vi "microspec_validating_v9.vi"() -> ()   [LabVIEW 2013]
uses:
  <vilib>/Instr/_visa.llb/VISA Configure Serial Port (Instr).vi
  <vilib>/Utility/file.llb/Write To Spreadsheet File (string).vi
panel:
  in  "Path":path
  in  "intergration time":dbl=54.0 caption="sensor\nintergration time (us)" min=54.0 max=5000000.0 step=100.0
  in  "?":T1(tab)=enum."measuring sequence"
  out "radiometer data file path":path
  in  "Runname":string
  out "Sensor_name":string="ILT1400"
  out "Radiometer Average":dbl
  in  "Delay":dbl=1.0
  in  "Step":dbl=1.0
  in  "Stop Wl":dbl=900.0 min=0.0 max=5000.0 step=100.0
  in  "Start Wl":dbl=300.0 min=0.0 max=5000.0 step=100.0
  in  "mean_number":i32=1 caption="Mean Number"
  out "Current Wavelength":dbl
  out "XY-Graph 2":cluster{"Y":dbl[], "Y":dbl[]}[](graph)
  in  "run 5":bool
  out "sectrometer data file path":path
  in  "save data":bool
  in  "reset with every wavelength?":bool caption="reset with new run?"
  in  "Delay":dbl=1.0
  in  "Step":dbl=10.0
  in  "Stop Wl":dbl=900.0 min=0.0 max=5000.0 step=100.0
  out "Current Wavelength":dbl
  in  "Start Wl 2":dbl=300.0 min=0.0 max=5000.0 step=10.0
  in  "Sensor":string(combo)="C12880MA_15B00040"
  in  "run 2":bool
  in  "Set Runs":i32=1
  out "Current Run":i32
  in  "stop runs":bool
  out "raw_data":cluster{"Y":dbl[], "Y":dbl[]}[](graph) caption="raw data"
  out "raw_data 2":cluster{"Y":dbl[], "Y":dbl[]}[](graph) caption="raw data"
  in  "Stopp":bool
  out "System Setup":i32
  out "DLL Version":string
  out "Get Version":i32
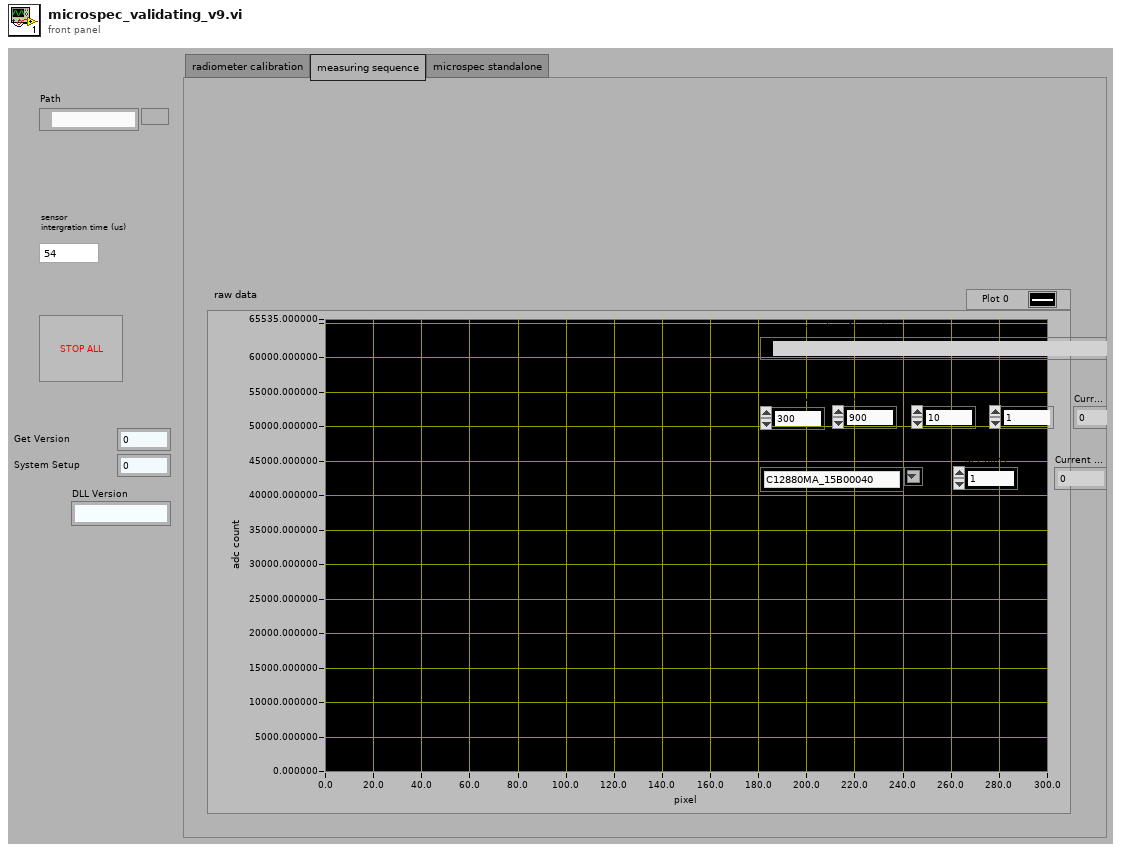
[diagram p1: front panel]
types:
  T1 = enum32{"radiometer calibration", "measuring sequence", "microspec standalone"}
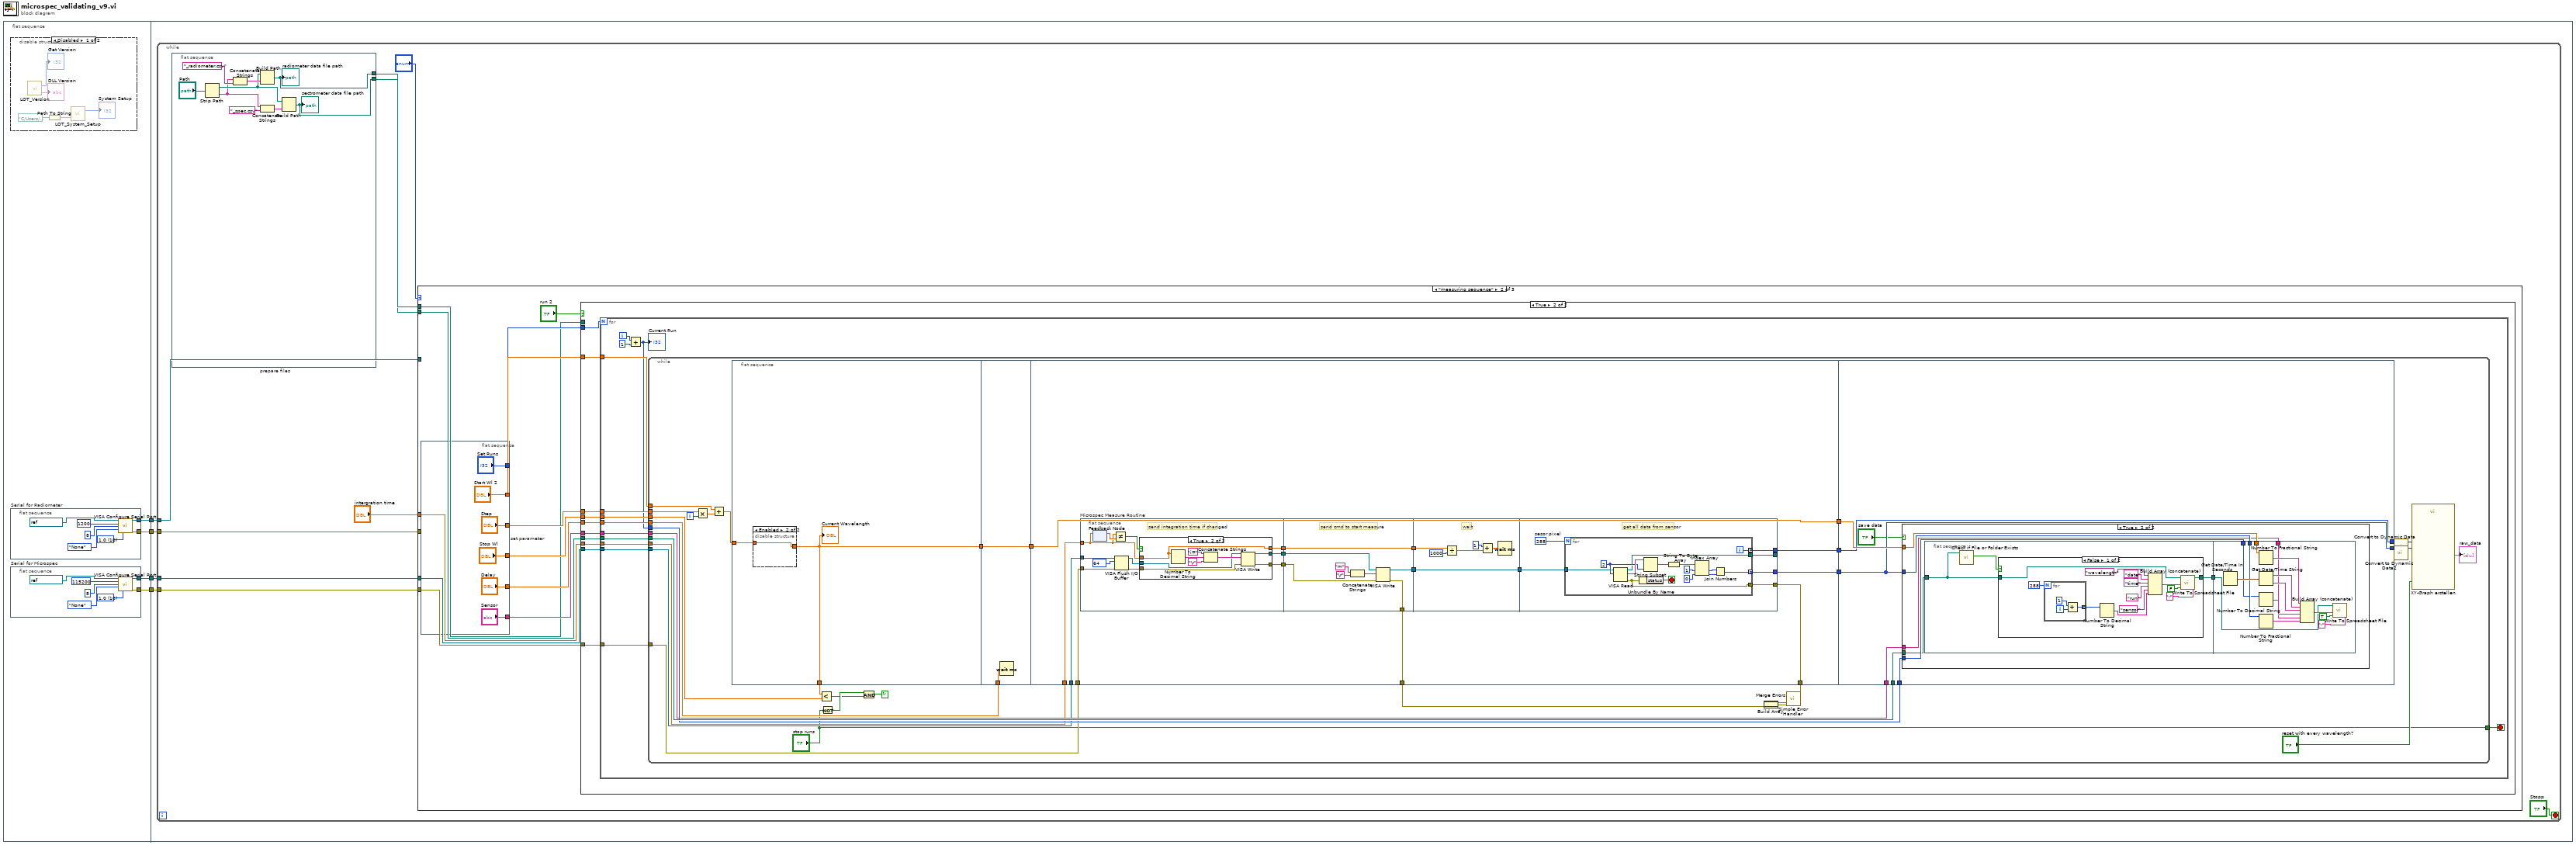
[diagram p0: block diagram]
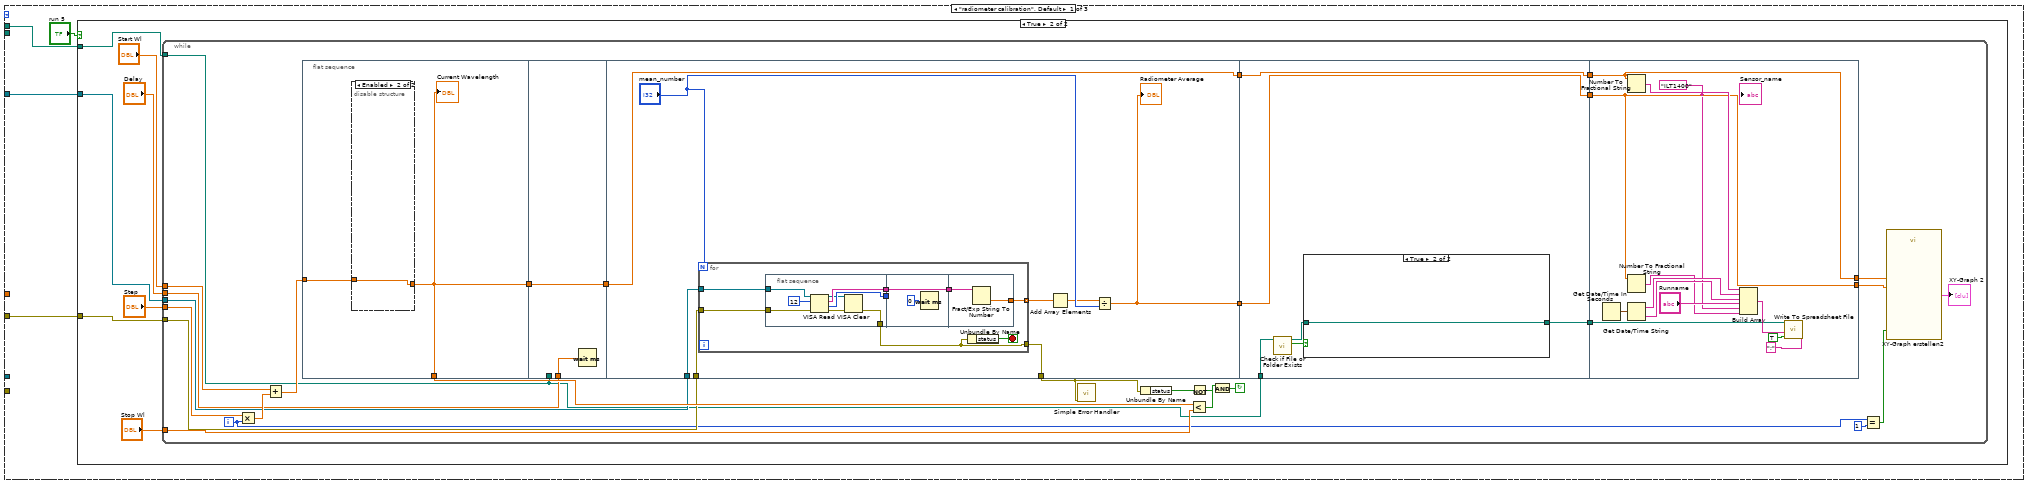
[diagram p3: hidden frame]
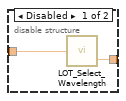
[diagram p5: hidden frame]
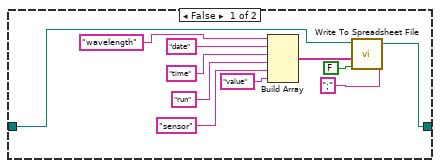
[diagram p6: hidden frame]
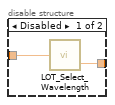
[diagram p8: hidden frame]
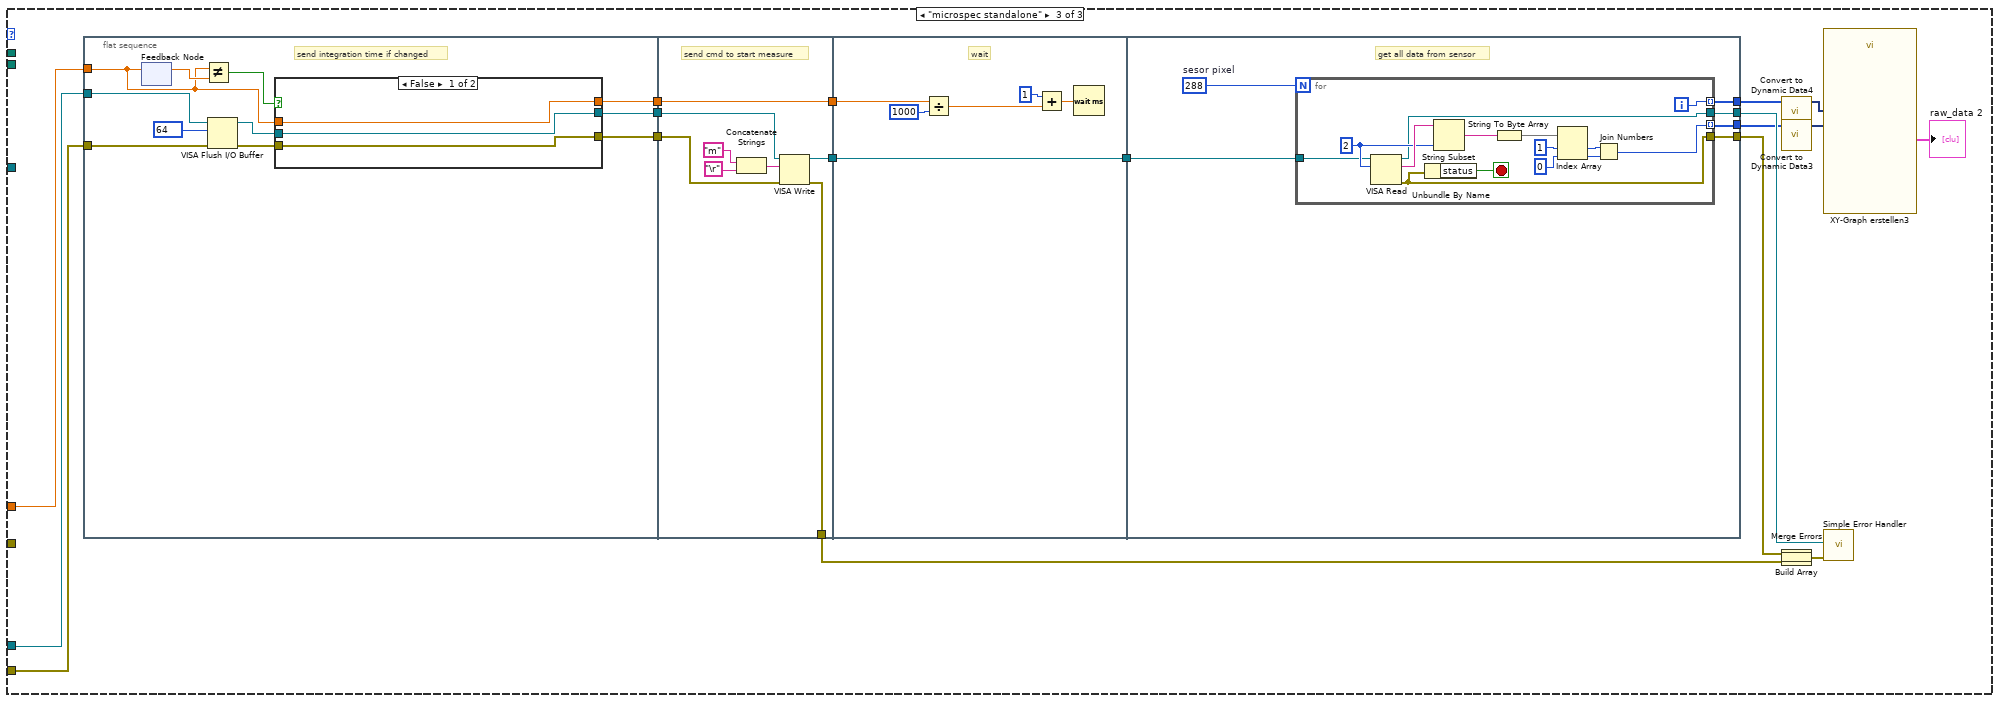
[diagram p12: hidden frame]
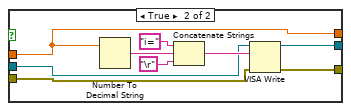
[diagram p13: hidden frame]
diagram:
  n1 = flat-sequence {
    tunnel: [w8] -> w4
    tunnel: [w7] -> w3
    tunnel: [w6] -> w2
    tunnel: [w5] -> w1
    tunnel: w4 -> [w31]
    tunnel: w3 -> [w30]
    tunnel: w2 -> [w29]
    tunnel: w1 -> [w28]
    frame #0 {
      # "Configuration"
      n2 = disable-structure shown="Disabled" {
        frame Disabled {
          n3 = call "LOT_Version.vi"() -> ("Version"=→"DLL Version":string, "Get Version"=→"Get Version":i32)
          n4 = Path To String(path=path "C:/Users/Public/Documents/LOT/Monochromator Control/Configurations/LOT_MSH-300_SN16578.xml" ("Configuration File")) -> (string=w25:string)
          n5 = call "LOT_System_Setup.vi"("CFG File Path"=w25) -> ("Error Code"=→"System Setup":i32)  [unwired: 2 in]
        }
        frame Enabled {
        }
      }
      n6 = flat-sequence "Serial for Radiometer" {
        tunnel: [w15] -> w6
        tunnel: [w14] -> w5
        frame #0 {
          w10 = u16 10 items=["1.0"=10, "1.5"=15, "2.0"=20] ("stop bits (10: 1 bit)")
          n7 = call-poly "VISA Configure Serial Port"("VISA resource name"=refnum<visa-resource-name> "COM4", "baud rate (9600)"=u32 1200, "data bits (8)"=u16 8, "parity (0:none)"=enum16{"None", "Odd", "Even", "Mark", "Space"}."None", "stop bits (10: 1 bit)"=w10) -> ("VISA resource name out"=w14:refnum<visa-resource-name>, "error out"=w15:errorcluster)  [unwired: 9 in]
        }
      }
      n8 = flat-sequence "Serial for Microspec" {
        tunnel: [w22] -> w8
        tunnel: [w21] -> w7
        frame #0 {
          w17 = u16 10 items=["1.0"=10, "1.5"=15, "2.0"=20] ("stop bits (10: 1 bit)")
          n9 = call-poly "VISA Configure Serial Port"("VISA resource name"=refnum<visa-resource-name> "COM11", "baud rate (9600)"=u32 115200, "data bits (8)"=u16 8, "parity (0:none)"=enum16{"None", "Odd", "Even", "Mark", "Space"}."None", "stop bits (10: 1 bit)"=w17) -> ("VISA resource name out"=w22:refnum<visa-resource-name>, "error out"=w21:errorcluster)  [unwired: 9 in]
        }
      }
    }
    frame #1 {
      n10 = while {
        tunnel: w31 -> [w38]
        tunnel: w30 -> [w37]
        tunnel: w29 -> [w36]
        tunnel: w28 -> [w35]
        stop <- "Stopp" stop-if-true
        n11 = flat-sequence "prepare files" {
          tunnel: [w41] -> w32
          tunnel: [w42] -> w33
          frame #0 {
            n12 = Strip Path(path="Path") -> (stripped path=w44:path, name=w43:string)
            n13 = Concatenate Strings(w43, "_radiometer.csv") -> (w45:string)
            n14 = Build Path(base path=w44, name or relative path=w45) -> (appended path=w42:path)
            "radiometer data file path" <- w42
            n15 = Concatenate Strings(w43, "_spec.csv") -> (w47:string)
            n16 = Build Path(base path=w44, name or relative path=w47) -> (appended path=w41:path)
            "sectrometer data file path" <- w41
          }
        }
        n17 = case shown="\"measuring sequence\"" "?" {
          tunnel: w32 -> [_ w165 _]
          tunnel: w38 -> [_ w164 w372]
          tunnel: w37 -> [_ w163 w371]
          tunnel: w36 -> [w52 _ _]
          tunnel: w35 -> [w51 _ _]
          tunnel: "intergration time" -> [_ w162 w370]
          tunnel: w33 -> [w50 w155 _]
          frame "radiometer calibration", Default {
            n18 = case shown="True" "run 5" {
              tunnel: w50 -> [_ w56]
              tunnel: w52 -> [_ w55]
              tunnel: w51 -> [_ w54]
              frame False {
              }
              frame True {
                n19 = while {
                  tunnel: "Step" -> [w88]
                  tunnel: "Start Wl" -> [w86]
                  tunnel: "Stop Wl" -> [w85]
                  tunnel: "Delay" -> [w81]
                  tunnel: w56 -> [w67]
                  tunnel: w54 -> [w80]
                  tunnel: w55 -> [w79]
                  i -> [w75]
                  stop <- w62 continue-if-true
                  n20 = Multiply(x=w88, y=w75) -> (x*y=w87:dbl)
                  n21 = Add(x=w86, y=w87) -> (x+y=w84:dbl)
                  n22 = flat-sequence {
                    tunnel: w84 -> [w90]
                    tunnel: [w89] -> w83
                    tunnel: [w89] -> w82
                    tunnel: w67 -> [_]
                    tunnel: w82 -> [w94]
                    tunnel: w81 -> [w95]
                    tunnel: [w94] -> w78
                    tunnel: w80 -> [w103]
                    tunnel: w79 -> [w102]
                    tunnel: w78 -> [w101]
                    tunnel: [w101] -> w71
                    tunnel: [w99] -> w69
                    tunnel: [w96] -> w61
                    tunnel: w71 -> [w129]
                    tunnel: [w129] -> w70
                    tunnel: w69 -> [w128]
                    tunnel: [w128] -> w68
                    tunnel: w67 -> [w126]
                    tunnel: [w127] -> w66
                    tunnel: [w145] -> w72
                    tunnel: [w146] -> w76
                    tunnel: w70 -> [w146]
                    tunnel: w68 -> [w145]
                    tunnel: w66 -> [w148]
                    frame #0 {
                      n23 = disable-structure shown="Enabled" {
                        disable-tunnel: w90 -> [w92 w93]
                        disable-tunnel: [w91 w93] -> w89
                        frame Disabled {
                          n24 = call "LOT_Select_Wavelength.vi"("Input Wavelength"=w92) -> ("Current Wavelength"=w91:dbl)  [unwired: 1 out]
                        }
                        frame Enabled {
                        }
                      }
                      "Current Wavelength" <- w89
                    }
                    frame #1 {
                      n25 = Wait (ms)(milliseconds to wait=w95) -> ()  [unwired: 1 out]
                    }
                    frame #2 {
                      n26 = for {
                        N: "mean_number" -> [_]
                        tunnel: w103 -> [w108]
                        tunnel: w102 -> [w107]
                        tunnel: [w106] -> w97 mode=indexing
                        tunnel: [w105] -> w96
                        stop <- w104 stop-if-true
                        n27 = flat-sequence {
                          tunnel: [w116] -> w111
                          tunnel: w108 -> [w119]
                          tunnel: w107 -> [w118]
                          tunnel: [w115] -> w110
                          tunnel: [w112] -> w105
                          tunnel: w111 -> [w121]
                          tunnel: [w121] -> w109
                          tunnel: w110 -> [_]
                          tunnel: w109 -> [w122]
                          tunnel: [w123] -> w106
                          frame #0 {
                            n28 = VISA Read(VISA resource name=w119, byte count=12, error in (no error)=w118) -> (VISA resource name out=w113:refnum<visa-resource-name>, read buffer=w116:string, return count=w115:u32, error out=w114:errorcluster)
                            n29 = VISA Clear(VISA resource name=w113, error in (no error)=w114) -> (error out=w112:errorcluster)  [unwired: 1 out]
                          }
                          frame #1 {
                            n30 = Wait (ms)(milliseconds to wait=u32 0 ("Zu wartende ms")) -> ()  [unwired: 1 out]
                          }
                          frame #2 {
                            n31 = Fract/Exp String To Number(string=w122) -> (number=w123:dbl)  [unwired: 3 in, 1 out]
                          }
                        }
                        n32 = Unbundle By Name(w105) -> ("status"=w104:bool)
                      }
                      n33 = Add Array Elements(numeric array=w97) -> (sum=w98:dbl)
                      n34 = Divide(x=w98, y="mean_number") -> (x/y=w99:dbl)
                      "Radiometer Average" <- w99
                    }
                    frame #3 {
                      n35 = call <vilib>:"Check if File or Folder Exists.vi"("path"=w126) -> ("file or folder exists?"=w125:bool, "dup path"=w124:path)  [unwired: 8 in, 1 out]
                      n36 = case shown="True" w125 {
                        tunnel: w124 -> [w138 w141]
                        tunnel: [w131 w141] -> w127
                        frame False {
                          n37 = Build Array("wavelength", "date" ("Element"), "time" ("Element"), "run" ("Element"), "sensor" ("Element"), "value") -> (w140:string[])
                          n38 = call-poly <vilib>:"Write To Spreadsheet File.vi"("delimiter (\\t)"=";", "append to file? (new file:F)"=FALSE, "1D data"=w140, "file path (dialog if empty)"=w138) -> ("new file path (Not A Path if cancelled)"=w131:path)  [unwired: 4 in]
                        }
                        frame True {
                        }
                      }
                    }
                    frame #4 {
                      w143 = "ILT1400" ("Sensor_name")
                      n39 = Get Date/Time In Seconds() -> (seconds since 1Jan1904=w153:timestamp)
                      n40 = Number To Fractional String(number=w146) -> (F-format string=w154:string)  [unwired: 3 in]
                      n41 = Number To Fractional String(number=w145) -> (F-format string=w142:string)  [unwired: 3 in]
                      n42 = Get Date/Time String(seconds (now)=w153) -> (date string=w152:string, time string=w151:string)  [unwired: 2 in]
                      n43 = Build Array(w154, w152, w151, "Runname", w143, w142) -> (w150:string[])
                      n44 = call-poly <vilib>:"Write To Spreadsheet File.vi"("delimiter (\\t)"=";", "append to file? (new file:F)"=TRUE, "1D data"=w150, "file path (dialog if empty)"=w148) -> ()  [unwired: 4 in, 1 out]
                      "Sensor_name" <- w143
                    }
                  }
                  n45 = call <vilib>:"Simple Error Handler.vi"("error in (no error)"=w61) -> ()  [unwired: 4 in, 5 out]
                  n46 = Unbundle By Name(w61) -> ("status"=w63:bool)
                  n47 = Less?(x=w83, y=w85) -> (x < y?=w65:bool)
                  n48 = Not(x=w63) -> (.not. x?=w64:bool)
                  n49 = And(x=w65, y=w64) -> (x .and. y?=w62:bool)
                  n50 = Equal?(x=w75, y=1) -> (x = y?=w73:bool)
                  n51 = call "XY-Graph erstellen2"("Reset"=w73, "Y Input"=w72, "X Input"=w76) -> ("XY Graph"=→"XY-Graph 2":cluster{"Y":dbl[], "Y":dbl[]}[])  [unwired: 7 in, 1 out]
                }
              }
            }
          }
          frame "measuring sequence" {
            n52 = flat-sequence "set parameter" {
              tunnel: ["Sensor"] -> w161
              tunnel: ["Delay"] -> w160
              tunnel: ["Step"] -> w159
              tunnel: ["Stop Wl"] -> w158
              tunnel: ["Start Wl 2"] -> w157
              tunnel: ["Set Runs"] -> w156
              frame #0 {
              }
            }
            n53 = case shown="True" "run 2" {
              tunnel: w165 -> [_ w173]
              tunnel: w161 -> [_ w182]
              tunnel: w156 -> [_ w181]
              tunnel: w164 -> [_ w180]
              tunnel: w163 -> [_ w179]
              tunnel: w160 -> [_ w178]
              tunnel: w158 -> [_ w177]
              tunnel: w159 -> [_ w176]
              tunnel: w157 -> [_ w175]
              tunnel: w162 -> [_ w174]
              tunnel: w155 -> [_ _]
              frame False {
              }
              frame True {
                n54 = for {
                  N: w181 -> [_]
                  tunnel: w173 -> [w195]
                  tunnel: w182 -> [w194]
                  tunnel: w180 -> [w193]
                  tunnel: w179 -> [w192]
                  tunnel: w178 -> [w191]
                  tunnel: w177 -> [w190]
                  tunnel: w176 -> [w189]
                  tunnel: w175 -> [w188]
                  tunnel: w174 -> [w187]
                  i -> [w186]
                  stop <- w183 stop-if-true
                  n55 = Add(x=w186, y=1) -> (x+y=w185:i32)
                  "Current Run" <- w185
                  n56 = while {
                    tunnel: w195 -> [w226]
                    tunnel: w185 -> [w225]
                    tunnel: w194 -> [w221]
                    tunnel: w193 -> [w219]
                    tunnel: w192 -> [w218]
                    tunnel: w191 -> [w209]
                    tunnel: w190 -> [w207]
                    tunnel: w189 -> [w206]
                    tunnel: w188 -> [w205]
                    tunnel: w187 -> [w204]
                    tunnel: ["stop runs"] -> w183
                    i -> [w223]
                    stop <- w198 continue-if-true
                    n57 = Multiply(x=w206, y=w223) -> (x*y=w228:dbl)
                    n58 = Add(x=w205, y=w228) -> (x+y=w227:dbl)
                    n59 = flat-sequence {
                      tunnel: w227 -> [w230]
                      tunnel: [w229] -> w224
                      tunnel: [w229] -> w208
                      tunnel: w224 -> [w234]
                      tunnel: w209 -> [w235]
                      tunnel: [w234] -> w212
                      tunnel: [w238] -> w220
                      tunnel: w219 -> [w242]
                      tunnel: w218 -> [w243]
                      tunnel: [w241] -> w216
                      tunnel: [w240] -> w215
                      tunnel: [w239] -> w214
                      tunnel: w212 -> [w238]
                      tunnel: w204 -> [w237]
                      tunnel: [w236] -> w203
                      tunnel: w226 -> [w313]
                      tunnel: w220 -> [w312]
                      tunnel: w225 -> [w311]
                      tunnel: [w309] -> w210
                      tunnel: w221 -> [w310]
                      tunnel: w214 -> [w309]
                      tunnel: w203 -> [w308]
                      tunnel: [w308] -> w202
                      frame #0 {
                        # "set wavelength"
                        n60 = disable-structure shown="Enabled" {
                          disable-tunnel: w230 -> [w232 w233]
                          disable-tunnel: [w231 w233] -> w229
                          frame Disabled {
                            n61 = call "LOT_Select_Wavelength.vi"("Input Wavelength"=w232) -> ("Current Wavelength"=w231:dbl)  [unwired: 1 out]
                          }
                          frame Enabled {
                          }
                        }
                        "Current Wavelength" <- w229
                      }
                      frame #1 {
                        # "wait"
                        n62 = Wait (ms)(milliseconds to wait=w235) -> ()  [unwired: 1 out]
                      }
                      frame #2 {
                        n63 = flat-sequence "Microspec Measure Routine" {
                          tunnel: w242 -> [w251]
                          tunnel: w243 -> [w260]
                          tunnel: [w255] -> w249
                          tunnel: [w254] -> w248
                          tunnel: [w253] -> w247
                          tunnel: w237 -> [w250]
                          tunnel: [w277] -> w246
                          tunnel: [w276] -> w240
                          tunnel: w249 -> [w274]
                          tunnel: w248 -> [w275]
                          tunnel: w247 -> [w273]
                          tunnel: [w273] -> w245
                          tunnel: w246 -> [w282]
                          tunnel: [w282] -> w244
                          tunnel: w245 -> [w281]
                          tunnel: w244 -> [w292]
                          tunnel: [w291] -> w239
                          tunnel: [w290] -> w236
                          tunnel: [w288] -> _
                          tunnel: [w287] -> w241
                          frame #0 {
                            # "send integration time if changed"
                            n64 = feedback-in #1(w250) -> ()
                            n65 = feedback #1() -> (w259:dbl)  [unwired: 1 in]
                            n66 = Not Equal?(x=w250, y=w259) -> (x != y?=w258:bool)
                            n67 = VISA Flush I/O Buffer(VISA resource name=w251, mask (16)=64, error in (no error)=w260) -> (VISA resource name out=w257:refnum<visa-resource-name>, error out=w256:errorcluster)
                            n68 = case shown="True" w258 {
                              tunnel: w257 -> [w262 w268]
                              tunnel: w256 -> [w261 w267]
                              tunnel: [w261 w266] -> w255
                              tunnel: [w262 w265] -> w254
                              tunnel: w250 -> [w263 w264]
                              tunnel: [w263 w264] -> w253
                              frame False {
                              }
                              frame True {
                                n69 = Number To Decimal String(number=w264) -> (decimal integer string=w271:string)  [unwired: 1 in]
                                n70 = Concatenate Strings("i=", w271, "\r") -> (w269:string)
                                n71 = VISA Write(VISA resource name=w268, write buffer=w269, error in (no error)=w267) -> (VISA resource name out=w265:refnum<visa-resource-name>, error out=w266:errorcluster)  [unwired: 1 out]
                              }
                            }
                          }
                          frame #1 {
                            # "send cmd to start measure"
                            n72 = Concatenate Strings("m", "\r") -> (w278:string)
                            n73 = VISA Write(VISA resource name=w275, write buffer=w278, error in (no error)=w274) -> (VISA resource name out=w277:refnum<visa-resource-name>, error out=w276:errorcluster)  [unwired: 1 out]
                          }
                          frame #2 {
                            # "wait"
                            n74 = Divide(x=w281, y=u32 1000 ("Zu wartende ms")) -> (x/y=w283:dbl)
                            n75 = Add(x=u32 1 ("Zu wartende ms"), y=w283) -> (x+y=w285:dbl)
                            n76 = Wait (ms)(milliseconds to wait=w285) -> ()  [unwired: 1 out]
                          }
                          frame #3 {
                            w289 = 288  # sesor pixel
                            # "get all data from sensor"
                            n77 = for {
                              N: w289 -> [_]
                              tunnel: w292 -> [w296]
                              tunnel: [w298] -> w291 mode=indexing
                              tunnel: [w297] -> w290 mode=indexing
                              tunnel: [w294] -> w288
                              tunnel: [w293] -> w287
                              i -> [w297]
                              stop <- w295 stop-if-true
                              w305 = 2
                              n78 = VISA Read(VISA resource name=w296, byte count=w305) -> (VISA resource name out=w294:refnum<visa-resource-name>, read buffer=w306:string, error out=w293:errorcluster)  [unwired: 1 in, 1 out]
                              n79 = Unbundle By Name(w293) -> ("status"=w295:bool)
                              n80 = String Subset(string=w306, length (rest)=w305) -> (substring=w304:string)  [unwired: 1 in]
                              n81 = String To Byte Array(string=w304) -> (unsigned byte array=w303:u8[])
                              n82 = Index Array(array=w303, index #1=1, index #2=0) -> (element #1=w299:u8, element #2=w300:u8)
                              n83 = Join Numbers(hi=w299, lo=w300) -> ((hi.lo)=w298:u16)
                            }
                          }
                        }
                      }
                      frame #3 {
                        n84 = case shown="True" "save data" {
                          tunnel: w313 -> [_ w316]
                          tunnel: w312 -> [_ w318]
                          tunnel: w311 -> [_ w317]
                          tunnel: w309 -> [_ w319]
                          tunnel: w310 -> [_ w315]
                          frame False {
                          }
                          frame True {
                            n85 = flat-sequence {
                              tunnel: w316 -> [w322]
                              tunnel: [w320] -> w314
                              tunnel: w319 -> [w346]
                              tunnel: w318 -> [w345]
                              tunnel: w317 -> [w344]
                              tunnel: w315 -> [w342]
                              tunnel: w314 -> [w340]
                              frame #0 {
                                n86 = call <vilib>:"Check if File or Folder Exists.vi"("path"=w322) -> ("file or folder exists?"=w321:bool)  [unwired: 8 in, 2 out]
                                n87 = case shown="False" w321 {
                                tunnel: w322 -> [w326 w339]
                                tunnel: [w323 w339] -> w320
                                frame False {
                                n88 = for {
                                N: 288 -> [_]
                                tunnel: [w336] -> w329 mode=indexing
                                i -> [w338]
                                n89 = Add(x=1, y=w338) -> (x+y=w336:i32)
                                }
                                n90 = Number To Decimal String(number=w329) -> (decimal integer string=w331:string[])  [unwired: 1 in]
                                n91 = Build Array (concatenate)("wavelength", "date" ("Element"), "time" ("Element"), "run" ("Element"), "sensor" ("Element"), w331) -> (w335:string[])
                                n92 = call-poly <vilib>:"Write To Spreadsheet File.vi"("delimiter (\\t)"=";", "append to file? (new file:F)"=FALSE, "1D data"=w335, "file path (dialog if empty)"=w326) -> ("new file path (Not A Path if cancelled)"=w323:path)  [unwired: 4 in]
                                }
                                frame True {
                                }
                                }
                              }
                              frame #1 {
                                n93 = Get Date/Time In Seconds() -> (seconds since 1Jan1904=w348:timestamp)
                                n94 = Number To Fractional String(number=w345) -> (F-format string=w347:string)  [unwired: 3 in]
                                n95 = Get Date/Time String(seconds (now)=w348) -> (date string=w349:string, time string=w350:string)  [unwired: 2 in]
                                n96 = Number To Decimal String(number=w344) -> (decimal integer string=w343:string)  [unwired: 1 in]
                                n97 = Number To Fractional String(number=w346) -> (F-format string=w353:string[])  [unwired: 3 in]
                                n98 = Build Array (concatenate)(w347, w349, w350, w343, w342, w353) -> (w351:string[])
                                n99 = call-poly <vilib>:"Write To Spreadsheet File.vi"("delimiter (\\t)"=";", "append to file? (new file:F)"=TRUE, "1D data"=w351, "file path (dialog if empty)"=w340) -> ()  [unwired: 4 in, 1 out]
                              }
                            }
                          }
                        }
                      }
                    }
                    n100 = Less?(x=w208, y=w207) -> (x < y?=w199:bool)
                    n101 = Not(x="stop runs") -> (.not. x?=w200:bool)
                    n102 = And(x=w200, y=w199) -> (x .and. y?=w198:bool)
                    n103 = Build Array(w216, w215) -> (w196:errorcluster[])
                    n104 = Merge Errors(w196) -> (w217:errorcluster)
                    n105 = call <vilib>:"Simple Error Handler.vi"("error in (no error)"=w217) -> ()  [unwired: 4 in, 5 out]
                    n106 = call "Convert to Dynamic Data"("Array"=w202) -> ("Dynamic Data Type"=w211:dynamicdata)  [unwired: 3 in]
                    n107 = call "Convert to Dynamic Data2"("Array"=w210) -> ("Dynamic Data Type"=w213:dynamicdata)  [unwired: 3 in]
                    n108 = call "XY-Graph erstellen"("Reset"="reset with every wavelength?", "Y Input"=w213, "X Input"=w211) -> ("XY Graph"=→"raw_data":cluster{"Y":dbl[], "Y":dbl[]}[])  [unwired: 7 in, 1 out]
                  }
                }
              }
            }
          }
          frame "microspec standalone" {
            n109 = flat-sequence {
              tunnel: w372 -> [w382]
              tunnel: w371 -> [w383]
              tunnel: [w377] -> w369
              tunnel: [w376] -> w368
              tunnel: [w375] -> w367
              tunnel: w370 -> [w373]
              tunnel: [w400] -> w366
              tunnel: [w399] -> w362
              tunnel: w369 -> [w397]
              tunnel: w368 -> [w398]
              tunnel: w367 -> [w396]
              tunnel: [w396] -> w365
              tunnel: w366 -> [w405]
              tunnel: [w405] -> w364
              tunnel: w365 -> [w404]
              tunnel: w364 -> [w414]
              tunnel: [w415] -> w363
              tunnel: [w413] -> w356
              tunnel: [w412] -> w355
              tunnel: [w410] -> w360
              frame #0 {
                # "send integration time if changed"
                n110 = feedback-in #2(w373) -> ()
                n111 = feedback #2() -> (w381:dbl)  [unwired: 1 in]
                n112 = Not Equal?(x=w373, y=w381) -> (x != y?=w380:bool)
                n113 = VISA Flush I/O Buffer(VISA resource name=w382, mask (16)=64, error in (no error)=w383) -> (VISA resource name out=w379:refnum<visa-resource-name>, error out=w378:errorcluster)
                n114 = case shown="False" w380 {
                  tunnel: w379 -> [w385 w391]
                  tunnel: w378 -> [w384 w390]
                  tunnel: [w384 w389] -> w377
                  tunnel: [w385 w388] -> w376
                  tunnel: w373 -> [w386 w387]
                  tunnel: [w386 w387] -> w375
                  frame False {
                  }
                  frame True {
                    n115 = Number To Decimal String(number=w387) -> (decimal integer string=w394:string)  [unwired: 1 in]
                    n116 = Concatenate Strings("i=", w394, "\r") -> (w392:string)
                    n117 = VISA Write(VISA resource name=w391, write buffer=w392, error in (no error)=w390) -> (VISA resource name out=w388:refnum<visa-resource-name>, error out=w389:errorcluster)  [unwired: 1 out]
                  }
                }
              }
              frame #1 {
                # "send cmd to start measure"
                n118 = Concatenate Strings("m", "\r") -> (w401:string)
                n119 = VISA Write(VISA resource name=w398, write buffer=w401, error in (no error)=w397) -> (VISA resource name out=w400:refnum<visa-resource-name>, error out=w399:errorcluster)  [unwired: 1 out]
              }
              frame #2 {
                # "wait"
                n120 = Divide(x=w404, y=u32 1000 ("Zu wartende ms")) -> (x/y=w406:dbl)
                n121 = Add(x=u32 1 ("Zu wartende ms"), y=w406) -> (x+y=w408:dbl)
                n122 = Wait (ms)(milliseconds to wait=w408) -> ()  [unwired: 1 out]
              }
              frame #3 {
                w411 = 288  # sesor pixel
                # "get all data from sensor"
                n123 = for {
                  N: w411 -> [_]
                  tunnel: w414 -> [w419]
                  tunnel: [w418] -> w415
                  tunnel: [w421] -> w413 mode=indexing
                  tunnel: [w420] -> w412 mode=indexing
                  tunnel: [w416] -> w410
                  i -> [w420]
                  stop <- w417 stop-if-true
                  w428 = 2
                  n124 = VISA Read(VISA resource name=w419, byte count=w428) -> (VISA resource name out=w416:refnum<visa-resource-name>, read buffer=w429:string, error out=w418:errorcluster)  [unwired: 1 in, 1 out]
                  n125 = Unbundle By Name(w418) -> ("status"=w417:bool)
                  n126 = String Subset(string=w429, length (rest)=w428) -> (substring=w427:string)  [unwired: 1 in]
                  n127 = String To Byte Array(string=w427) -> (unsigned byte array=w426:u8[])
                  n128 = Index Array(array=w426, index #1=1, index #2=0) -> (element #1=w422:u8, element #2=w423:u8)
                  n129 = Join Numbers(hi=w422, lo=w423) -> ((hi.lo)=w421:u16)
                }
              }
            }
            n130 = call "Convert to Dynamic Data4"("Array"=w355) -> ("Dynamic Data Type"=w357:dynamicdata)  [unwired: 3 in]
            n131 = call "Convert to Dynamic Data3"("Array"=w356) -> ("Dynamic Data Type"=w358:dynamicdata)  [unwired: 3 in]
            n132 = Build Array(w363, w362) -> (w354:errorcluster[])
            n133 = Merge Errors(w354) -> (w361:errorcluster)
            n134 = call "XY-Graph erstellen3"("Y Input"=w358, "X Input"=w357) -> ("XY Graph"=→"raw_data 2":cluster{"Y":dbl[], "Y":dbl[]}[])  [unwired: 8 in, 1 out]
            n135 = call <vilib>:"Simple Error Handler.vi"("error source (\" \")"=w360, "error in (no error)"=w361) -> ()  [unwired: 3 in, 5 out]
          }
        }
      }
    }
  }
